vi "Run Player Bar.vi"(13 "IMAQ Display Refs":refnum<vi>[](array[refnum])) -> ()   [LabVIEW 2016]
uses:
  <vilib>/event_ctls.llb/lveventtype.ctl
panel:
  in  "Exit":bool
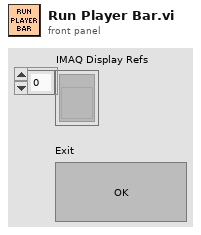
[diagram p1: front panel]
types:
  T1 = typedef "lveventtype.ctl" = enum32{"Null", "Timeout", "Annotation Menu Selection", "Annotation Menu Selection?", "App Instance Close", "App Instance Close?", "Autoscale Range Change", "Bookmark Info Change", "Cell Edit", "Cell Edit?", "Cursor Grab", "Cursor Grab?", "Cursor Menu Selection", "Cursor Menu Selection?", "Cursor Move", "Cursor Release", "Data Change", "Direction Change", "Display State Change", "Drag Ended", "Drag Enter", "Drag Leave", "Drag Over", "Drag Source Update", "Drag Starting", "Drag Starting?", "Drop", "Exec State Change", "Key Down", "Key Down?", "Key Repeat", "Key Repeat?", "Key Up", "Listbox Double Click", "Menu Activation?", "Menu Selection (App)", "Menu Selection? (App)", "Menu Selection (User)", "Mouse Down", "Mouse Down?", "Mouse Enter", "Mouse Leave", "Mouse Move", "Mouse Up", "Mouse Wheel", "NI Security User Change (App)", "Pane Size", "Panel Close", "Panel Close?", "Panel Resize", "Plot Attribute Change", "Scale Range Change", "Shortcut Menu Activation?", "Shortcut Menu Selection (App)", "Shortcut Menu Selection? (App)", "Shortcut Menu Selection (User)", "Tree Double Click", "Tree Drag", "Tree Drag?", "Tree Drop", "Tree Drop?", "Tree Item Close", "Tree Item Close?", "Tree Item Open", "Tree Item Open?", "User Event", "Value Change"}
  T2 = enum32{"Invalid", "Standard", "Closed", "Hidden", "Minimized", "Maximized"}
  T3 = enum32{"Bad", "Idle", "Run top level", "Running"}
  T4 = typedef "LVRectTypeDef.ctl" = cluster{"Left":i16, "Top":i16, "Right":i16, "Bottom":i16}
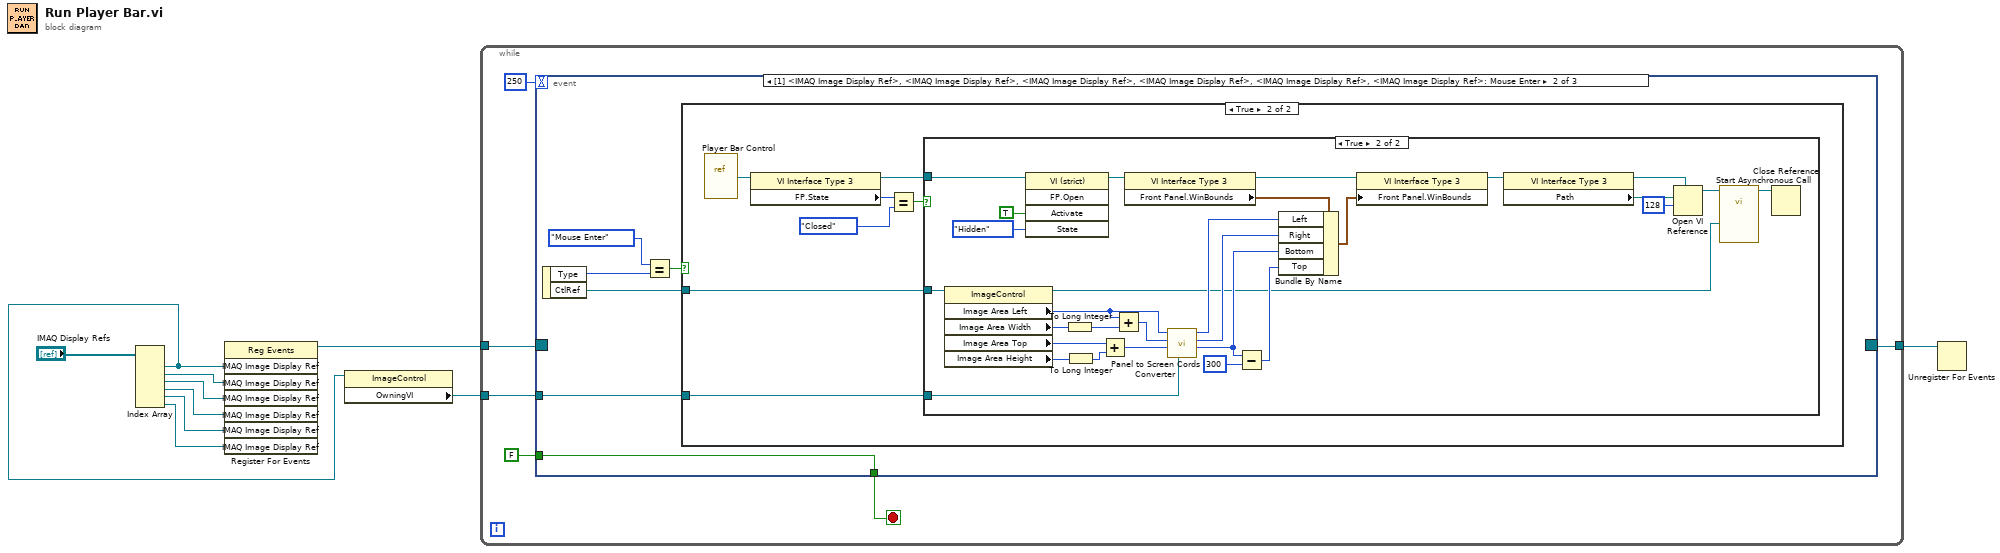
[diagram p0: block diagram]
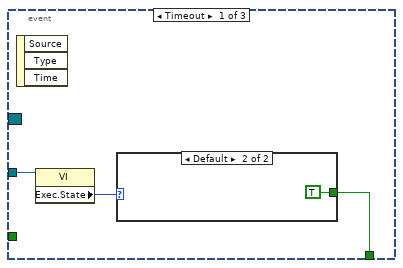
[diagram p2: hidden frame]
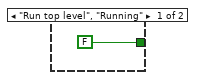
[diagram p3: hidden frame]
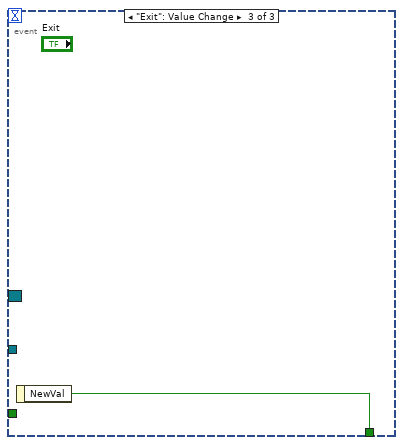
[diagram p6: hidden frame]
diagram:
  n1 = Index Array(array="IMAQ Display Refs") -> (element #1=w1:refnum<vi>, element #2=w6:refnum<vi>, element #3=w3:refnum<vi>, element #4=w4:refnum<vi>, element #5=w5:refnum<vi>, element #6=w2:refnum<vi>)  [unwired: 6 in]
  n2 = register-events(w1, w6, w3, w4, w5, w2) -> (reference out=w10:refnum<event-registration>)  [unwired: 2 in, 1 out]
  n3 = property class="ImageControl"(reference=w1) -> ("OwningVI"=w8:refnum<vi>)  [unwired: 1 in, 2 out]
  n4 = while {
    tunnel: w10 -> [w14]
    tunnel: [w13] -> w9
    tunnel: w8 -> [w11]
    stop <- w15 stop-if-true
    n5 = event shown="[1] <IMAQ Image Display Ref>, <IMAQ Image Display Ref>, <IMAQ Image Display Ref>, <IMAQ Image Display Ref>, <IMAQ Image Display Ref>, <IMAQ Image Display Ref>: Mouse Enter" {
      selector: w14 -> [_ _ _]
      dyn-events: [_ _ _] -> w13
      timeout: 250 -> [_ _ _]
      tunnel: FALSE -> [_ w27 _]
      tunnel: [w17 w27 w64] -> w15
      tunnel: w11 -> [w18 w22 _]
      event Timeout {
        n6 = event-data() -> ()  [unwired: 1 in, 3 out]
        n7 = property class="VI"(reference=w18) -> ("Exec.State"=w19:T3)  [unwired: 1 in, 2 out]
        n8 = case shown="Default" w19 {
          tunnel: [FALSE TRUE] -> w17
          frame "Run top level", "Running" {
          }
          frame Default {
          }
        }
      }
      event Mouse Enter {
        n9 = event-data() -> ("Type"=w25:T1, "CtlRef"=w23:refnum<vi>)  [unwired: 1 in]
        n10 = Equal?(x=lveventtype."Mouse Enter" ("Type"), y=w25) -> (x = y?=w24:bool)
        n11 = case shown="True" w24 {
          tunnel: w23 -> [_ w30]
          tunnel: w22 -> [_ w28]
          frame False {
          }
          frame True {
            n12 = vi-ref "Player Bar Control.vi"() -> (w29:refnum<vi>)
            n13 = property class="VI Interface Type 3"(reference=w29) -> (reference out=w32:refnum<vi>, "FP.State"=w34:T2)  [unwired: 1 in, 1 out]
            n14 = Equal?(x=w34, y=T2."Closed" ("Front Panel Window:State")) -> (x = y?=w31:bool)
            n15 = case shown="True" w31 {
              tunnel: w32 -> [_ w52]
              tunnel: w30 -> [_ w51]
              tunnel: w28 -> [_ w35]
              frame False {
              }
              frame True {
                n16 = property class="ImageControl"(reference=w51) -> (reference out=w36:refnum<vi>, "Image Area Left"=w44:i32, "Image Area Width"=w43:u32, "Image Area Top"=w39:i32, "Image Area Height"=w41:u32)  [unwired: 1 in, 1 out]
                n17 = invoke class="VI (strict)" method="FP.Open"(reference=w52, "Activate"=TRUE ("Activate?"), "State"=T2."Hidden") -> (reference out=w58:refnum<vi>)  [unwired: 2 in, 4 out]
                n18 = To Long Integer(number=w43) -> (32bit integer=w40:i32)
                n19 = To Long Integer(number=w41) -> (32bit integer=w37:i32)
                n20 = Add(x=w39, y=w37) -> (x+y=w38:i32)
                n21 = Add(x=w44, y=w40) -> (x+y=w42:i32)
                n22 = property class="VI Interface Type 3"(reference=w58) -> (reference out=w59:refnum<vi>, "Front Panel.WinBounds"=w60:T4)  [unwired: 1 in, 1 out]
                n23 = call "Panel to Screen Cords Converter.vi"("VI Ref"=w35, "Vertical FP 1"=w38, "Horizontal FP 2"=w42, "Horizontal FP 1"=w44) -> ("Vertical Screen 1"=w47:i16, "Horizontal Screen 2"=w45:i16, "Horizontal Screen 1"=w46:i16)  [unwired: 4 in, 1 out]
                n24 = Subtract(x=w47, y=i16 300) -> (x-y=w48:i16)
                n25 = Bundle By Name(cluster=w60, "Left"=w46, "Right"=w45, "Bottom"=w47, "Top"=w48) -> (w61:T4)
                n26 = property class="VI Interface Type 3"(reference=w59, "Front Panel.WinBounds"=w61) -> (reference out=w50:refnum<vi>)  [unwired: 1 in, 1 out]
                n27 = property class="VI Interface Type 3"(reference=w50) -> (reference out=w53:refnum<vi>, "Path"=w57:path)  [unwired: 1 in, 1 out]
                n28 = Open VI Reference(type specifier VI Refnum (for type only)=w53, vi path=w57, options=128) -> (vi reference=w55:refnum<vi>)  [unwired: 3 in, 1 out]
                n29 = call-by-ref "Start Asynchronous Call"(reference=w55, "Ctl Refnum 2"=w36) -> (reference out=w54:refnum<vi>)  [unwired: 16 in, 1 out]
                n30 = Close Reference(reference=w54) -> ()  [unwired: 1 in, 1 out]
              }
            }
          }
        }
      }
      event "Exit": Value Change {
        n31 = event-data() -> ("NewVal"=w64:bool)  [unwired: 1 in]
      }
    }
  }
  n32 = Unregister For Events(event registration refnum=w9) -> ()  [unwired: 1 in, 1 out]
